vi "restore permissions of RT images directory.vi"(11 "directory":path=path "C:/Program Files (x86)/National Instruments/RT Images") -> (0 "error out":errorcluster, 3 "permissions":i16 format="%o")   [LabVIEW 2013]
uses:
  file permissions action.ctl
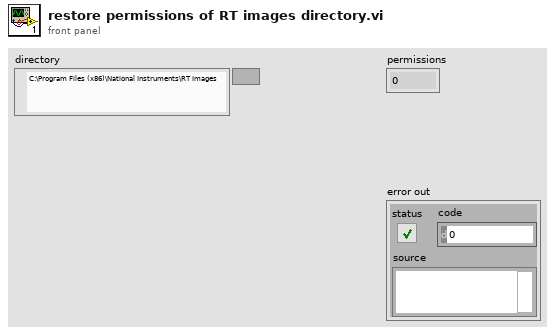
[diagram p1: front panel]
types:
  T1 = typedef "file permissions action.ctl" = enum16{"get", "set", "reset"}
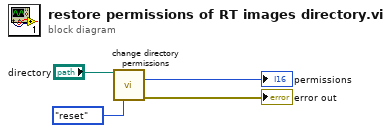
[diagram p0: block diagram]
diagram:
  n1 = call "change directory permissions.vi"("directory"="directory", "action (get)"=file_permissions_action."reset") -> ("permissions"=→"permissions":i16, "error out"=→"error out":errorcluster)  [unwired: 11 in, 1 out]
